vi "Create PathMsg.vi"(8 "error in (no error)":errorcluster, 10 "Message Data":path, 11 "Message Name":string) -> (0 "error out":errorcluster, 3 "PathMsg out":refnum<class "PathMsg.lvclass">)   [LabVIEW 2013, in "LapDog.Messaging.v3.NativeTypes.lvlib" / "PathMsg.lvclass"]
doc: "Returns a PathMsg object with the given name.\n\nThis method executes regardless of the error in state."
uses:
  PathMsg.lvclass
  LapDog.Messaging/Message/Message.lvclass
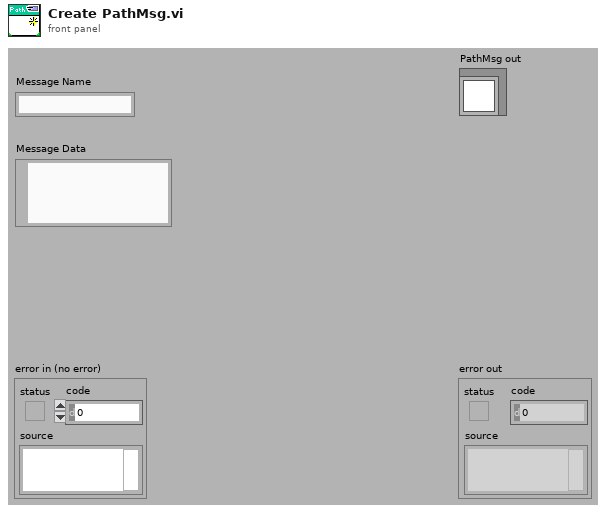
[diagram p1: front panel]
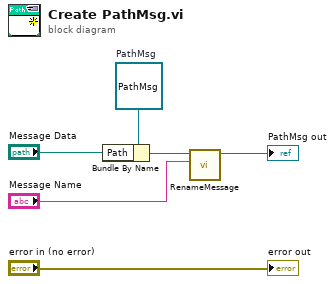
[diagram p0: block diagram]
diagram:
  w1 = refnum<class "PathMsg.lvclass"> refnum  # PathMsg
  n1 = Bundle By Name(cluster=w1, "Path"="Message Data") -> (w4:refnum<class "PathMsg.lvclass">)
  n2 = call "RenameMessage.vi"("Message Name"="Message Name", "Message in"=w4) -> ("Message out"=→"PathMsg out":refnum<class "PathMsg.lvclass">)  [unwired: 8 in, 1 out]
  "error out" <- "error in (no error)"
